vi "FuncTest.vi"() -> ()   [LabVIEW 2015]
panel:
  out "element 2":u8
  out "element":u8
  out "Numeric 3":i32
  out "Numeric 2":i32
  in  "stop":bool
  in  "Numeric":dbl format="%#_13g"
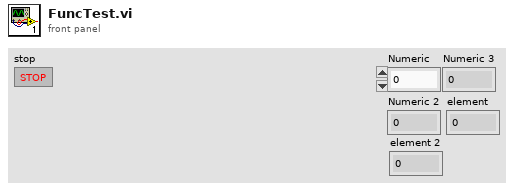
[diagram p1: front panel]
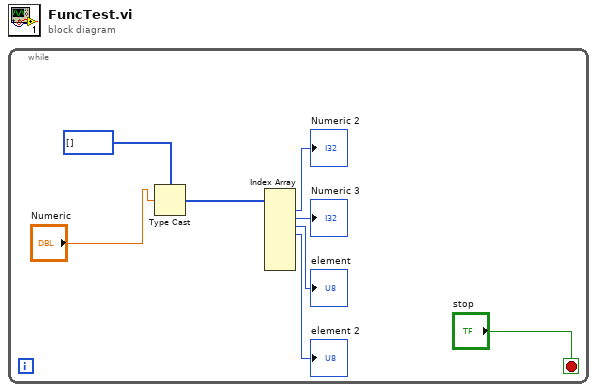
[diagram p0: block diagram]
diagram:
  n1 = while {
    stop <- "stop" stop-if-true
    n2 = Type Cast(type=u8[] [], x="Numeric") -> (*(type *) &x=w5:u8[])
    n3 = Index Array(array=w5) -> (element #1=→"Numeric 2":u8, element #2=→"Numeric 3":u8, element #3=→"element":u8, element #4=→"element 2":u8)  [unwired: 8 in, 4 out]
  }
